vi "Calculate Built Version.vi"(0 "VIP in":refnum<class "VIP.lvclass">, 11 "error in (no error)":errorcluster) -> (4 "VIP out":refnum<class "VIP.lvclass">, 15 "error out":errorcluster)   [LabVIEW 2017, in "CL_G3_VIComponentBuilder.lvlib" / "VIP.lvclass"]
doc: "Uses the VIPM API to calculate the built version of the export."
uses:
  VIP.lvclass
  C:/builds/Component BuilderBT/SrcDist/Exports/Exports/Export.lvclass
  Exports/Export.lvclass/Export.ctl
  Exports/Accessors/Read Built Export's Full Path.vi
  Exports/Accessors/Write Built Version.vi
  VIPM Utilities/CL_G3_VIPMUtilities.lvlib
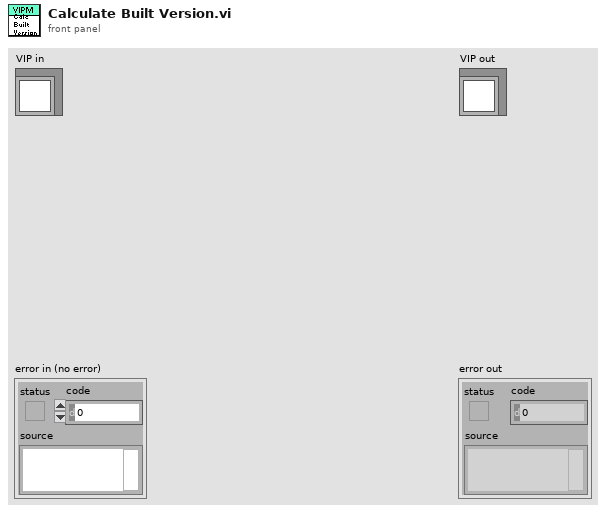
[diagram p1: front panel]
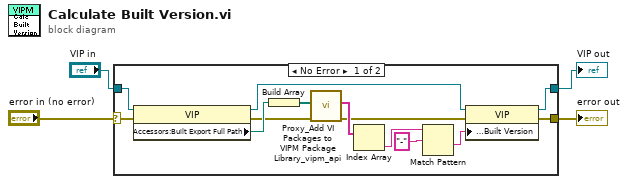
[diagram p0: block diagram]
diagram:
  n1 = case shown="No Error" "error in (no error)" {
    selector: "error in (no error)" -> [w17 w18]
    tunnel: "VIP in" -> [w7 w19]
    tunnel: [w6 w18] -> w2
    tunnel: [w5 w19] -> w1
    frame No Error {
      n2 = property class="VIP"(reference=w7, error in=w17) -> (reference out=w12:refnum<class "VIP.lvclass">, error out=w9:errorcluster, "Accessors:Built Export Full Path"=w13:path)
      n3 = Build Array(w13) -> (w16:path[])
      n4 = call "Proxy_Add VI Packages to VIPM Package Library_vipm_api.vi"("error in (no error)"=w9, "Packages to add to VIPM Library (vipc,vip,ogp)"=w16) -> ("error out"=w8:errorcluster, "Package Names Added"=w15:string[])  [unwired: 8 in]
      n5 = Index Array(array=w15) -> (element=w11:string)  [unwired: 1 in]
      n6 = Match Pattern(string=w11, regular expression="-") -> (after substring=w10:string)  [unwired: 1 in, 3 out]
      n7 = property class="VIP"(reference=w12, error in=w8, "Accessors:Built Version"=w10) -> (reference out=w5:refnum<class "VIP.lvclass">, error out=w6:errorcluster)
    }
    frame Error {
    }
  }
  "error out" <- w2
  "VIP out" <- w1
